vi "CreateHandle.vi"   [LabVIEW 2015]
uses:
  MvCameraControl.lvlib
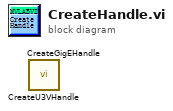
[diagram p0: block diagram]
diagram:
  n1 = call "CreateU3VHandle.vi"() -> ()  [unwired: 8 in, 3 out]
  n2 = call "CreateGigEHandle.vi"() -> ()  [unwired: 8 in, 3 out]
